vi "Choose Selected Control.vi"(11 "reference":refnum<vi>) -> (3 "appended array":refnum<vi>[](array[refnum]), 5 "Position":T1, 7 "Owner":refnum<vi>)   [LabVIEW 2015]
uses:
  <vilib>/Utility/miscctls.llb/LVPositionTypeDef.ctl
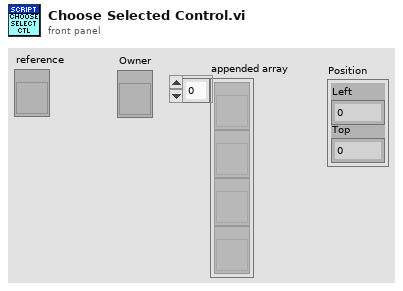
[diagram p1: front panel]
types:
  T1 = typedef "LVPositionTypeDef.ctl" = cluster{"Left":i32, "Top":i32}
  T2 = typedef "LVRectTypeDef.ctl" = cluster{"Left":i16, "Top":i16, "Right":i16, "Bottom":i16}
  T3 = typedef "LVPointTypeDef.ctl" = cluster{"Horizontal":i16, "Vertical":i16}
  T4 = cluster{refnum<vi>, "Position":cluster{"Width":dbl, "Height":dbl}}
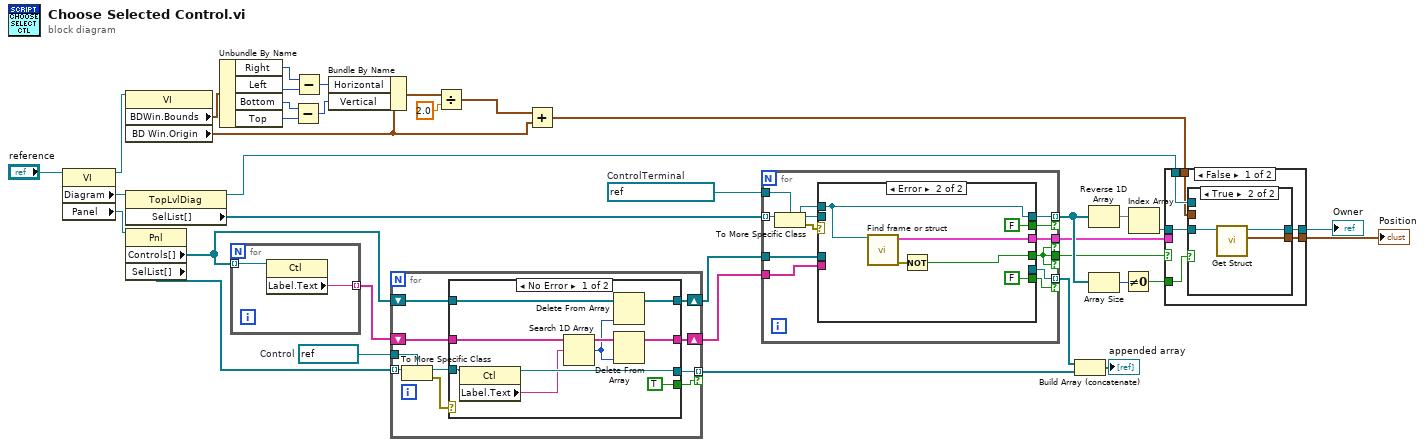
[diagram p0: block diagram]
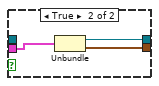
[diagram p3: hidden frame]
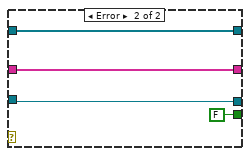
[diagram p4: hidden frame]
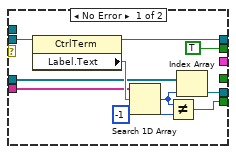
[diagram p5: hidden frame]
diagram:
  w30 = refnum<vi> refnum  # ControlTerminal
  w32 = refnum<vi> refnum  # Control
  n1 = property class="VI"(reference="reference") -> (reference out=w9:refnum<vi>, "Diagram"=w37:refnum<vi>, "Panel"=w36:refnum<vi>)  [unwired: 1 in, 1 out]
  n2 = property class="VI"(reference=w9) -> ("BDWin.Bounds"=w12:T2, "BD Win.Origin"=w5:T3)  [unwired: 1 in, 2 out]
  n3 = property class="TopLvlDiag"(reference=w37) -> (reference out=w8:refnum<vi>, "SelList[]"=w35:refnum<vi>[])  [unwired: 1 in, 1 out]
  n4 = property class="Pnl"(reference=w36) -> ("Controls[]"=w29:refnum<vi>[], "SelList[]"=w34:refnum<vi>[])  [unwired: 1 in, 2 out]
  n5 = Unbundle By Name(w12) -> ("Right"=w13:i16, "Left"=w14:i16, "Bottom"=w11:i16, "Top"=w17:i16)
  n6 = for {
    tunnel: w29 -> [w39] mode=indexing
    tunnel: [w38] -> w33 mode=indexing
    n7 = property class="Ctl"(reference=w39) -> ("Label.Text"=w38:string)  [unwired: 1 in, 2 out]
  }
  n8 = Subtract(x=w11, y=w17) -> (x-y=w16:i16)
  n9 = Subtract(x=w13, y=w14) -> (x-y=w15:i16)
  n10 = Bundle By Name(cluster=w5, "Horizontal"=w15, "Vertical"=w16) -> (w18:T3)
  n11 = for {
    tunnel: w34 -> [w49] mode=indexing
    tunnel: [w47] -> w26 mode=indexing if=w44
    tunnel: w32 -> [w46]
    shift-right: [w42] -> w31
    shift-left: w33 -> [w43]
    shift-right: [w40] -> w28
    shift-left: w29 -> [w41]
    n12 = To More Specific Class(target class=w46, reference=w49) -> (specific class reference=w48:refnum<vi>, error out=w45:errorcluster)  [unwired: 1 in]
    n13 = case shown="No Error" w45 {
      tunnel: w48 -> [w58 w61]
      tunnel: [w57 w61] -> w47
      tunnel: [TRUE FALSE] -> w44
      tunnel: w43 -> [w54 w60]
      tunnel: [w53 w60] -> w42
      tunnel: w41 -> [w52 w59]
      tunnel: [w50 w59] -> w40
      frame No Error {
        n14 = property class="Ctl"(reference=w58) -> (reference out=w57:refnum<vi>, "Label.Text"=w55:string)  [unwired: 1 in, 1 out]
        n15 = Search 1D Array(1D array=w54, element=w55) -> (index of element=w51:i32)  [unwired: 1 in]
        n16 = Delete From Array(array=w52, index=w51) -> (array with subset deleted=w50:refnum<vi>[])  [unwired: 1 in, 1 out]
        n17 = Delete From Array(array=w54, index=w51) -> (array with subset deleted=w53:string[])  [unwired: 1 in, 1 out]
      }
      frame Error {
      }
    }
  }
  n18 = Divide(x=w18, y=2.0) -> (x/y=w19:cluster{"Horizontal":dbl, "Vertical":dbl})
  n19 = Add(x=w19, y=w5) -> (x+y=w10:cluster{"Horizontal":dbl, "Vertical":dbl})
  n20 = for {
    tunnel: w35 -> [w66] mode=indexing
    tunnel: w30 -> [w67]
    tunnel: w28 -> [w72]
    tunnel: w31 -> [w63]
    tunnel: [w71] -> w27 mode=indexing if=w70
    tunnel: [w69] -> w4 mode=indexing if=w68
    tunnel: [w65] -> w3 if=w64
    tunnel: [w64] -> w2 if=w64
    n21 = To More Specific Class(target class=w67, reference=w66) -> (specific class reference=w73:refnum<vi>, error out=w74:errorcluster)  [unwired: 1 in]
    n22 = case shown="Error" w74 {
      tunnel: w73 -> [w84 _]
      tunnel: w63 -> [w82 _]
      tunnel: w72 -> [w81 _]
      tunnel: [w80 _] -> w71
      tunnel: [w77 FALSE] -> w70
      tunnel: [w76 w88] -> w69
      tunnel: [TRUE FALSE] -> w68
      tunnel: w66 -> [_ w88]
      tunnel: [_ w87] -> w65
      tunnel: [_ w86] -> w64
      frame No Error {
        n23 = property class="CtrlTerm"(reference=w84) -> (reference out=w76:refnum<vi>, "Label.Text"=w83:string)  [unwired: 1 in, 1 out]
        n24 = Search 1D Array(1D array=w82, element=w83) -> (index of element=w79:i32)  [unwired: 1 in]
        n25 = Not Equal?(x=w79, y=-1) -> (x != y?=w77:bool)
        n26 = Index Array(array=w81, index=w79) -> (element=w80:refnum<vi>)
      }
      frame Error {
        n27 = call <resource>:"Find frame or struct.vi"("GObj Refnum"=w88) -> ("error IO"=w85:errorcluster, "output cluster"=w87:T4)  [unwired: 9 in]
        n28 = Not(x=w85) -> (.not. x?=w86:bool)
      }
    }
  }
  n29 = Build Array (concatenate)(w27, w26) -> (→"appended array":refnum<vi>[])
  n30 = Reverse 1D Array(array=w4) -> (reversed array=w23:refnum<vi>[])
  n31 = Array Size(array=w4) -> (size(s)=w21:i32)
  n32 = Not Equal To 0?(x=w21) -> (x != 0?=w1:bool)
  n33 = Index Array(array=w23) -> (element=w22:refnum<vi>)  [unwired: 1 in]
  n34 = case shown="False" w2 {
    tunnel: w22 -> [w94 _]
    tunnel: [w93 w103] -> w6
    tunnel: w10 -> [w91 _]
    tunnel: [w92 w102] -> w7
    tunnel: w8 -> [w95 _]
    tunnel: w3 -> [_ w104]
    tunnel: w1 -> [w96 _]
    frame False {
      n35 = case shown="True" w96 {
        tunnel: [w98 w100] -> w93
        tunnel: w95 -> [w98 _]
        tunnel: w91 -> [w97 _]
        tunnel: [w97 w99] -> w92
        tunnel: w94 -> [_ w101]
        frame False {
        }
        frame True {
          n36 = call <resource>:"Get Struct.vi"("reference"=w101) -> ("Position"=w99:T1, "Gen Refnum"=w100:refnum<vi>)  [unwired: 9 in]
        }
      }
    }
    frame True {
      n37 = Unbundle(w104) -> (w103:refnum<vi>, "Position"=w102:cluster{"Width":dbl, "Height":dbl})
    }
  }
  "Position" <- w7
  "Owner" <- w6
